vi "path.vi"() -> ()   [LabVIEW 2018]
panel:
  in  "Path":path
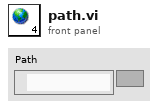
[diagram p1: front panel]
diagram:
